vi "Stalled.vi"(6 "Stall Time (ms)":u32=300, 7 "Model Name":T1=enum."W 601 FR RH Std", 9 "Max Run Current":dbl=10.0, 10 "millisecond timer value in":u32, 11 "Inputs":T2) -> (1 "Stalled":bool, 2 "millisecond timer value out":u32)   [LabVIEW 2017]
uses:
  controls/All Inputs.ctl
  controls/SACB DI.ctl
  controls/Model Name.ctl
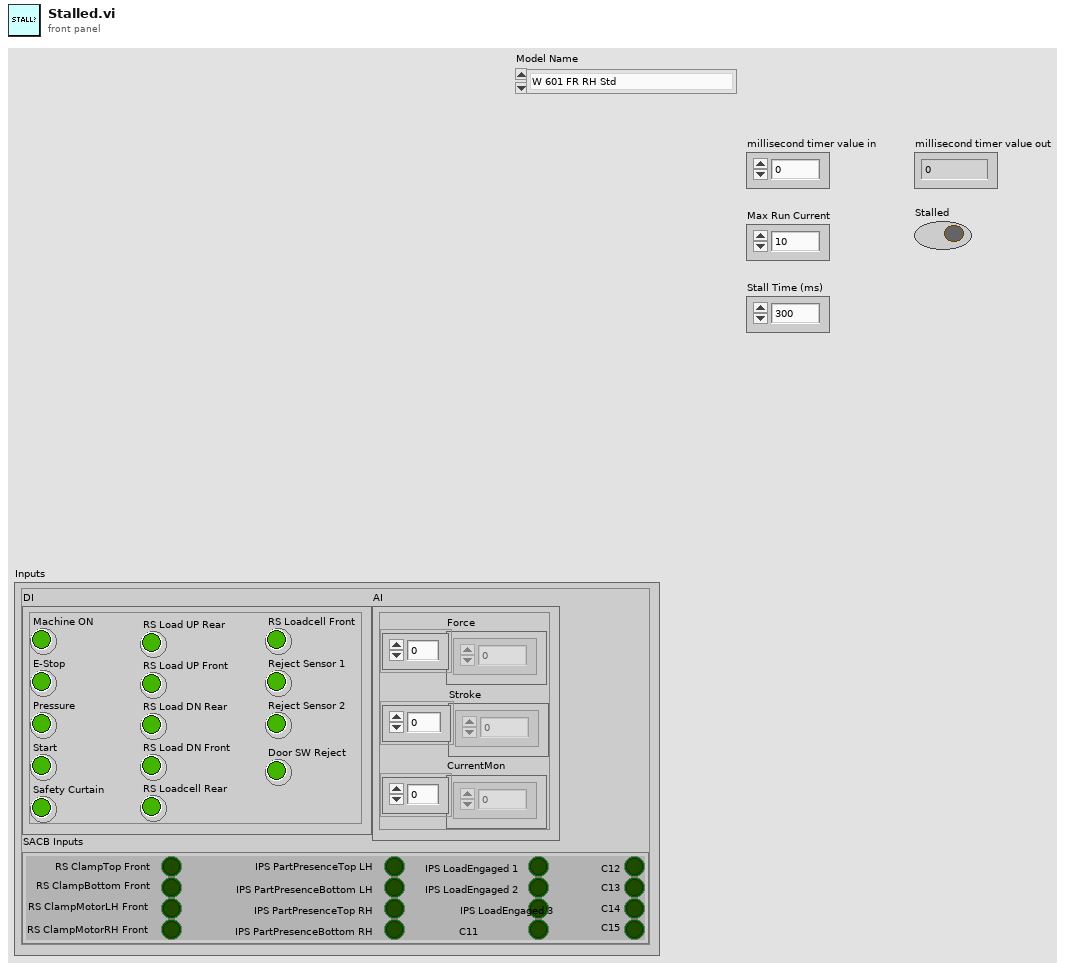
[diagram p1: front panel]
types:
  T1 = typedef "Model Name.ctl" = enum16{"W 501 FLH Std.", "W 501 FRH Std.", "W 601 FR RH Std", "W 601 FR LH Std", "W 601 RR RH Std", "W 601 RR LH Std", "W 601 FR RH AP", "W 601 FR LH AP", "W 601 RR RH AP", "W 601 RR LH AP"}
  T2 = typedef "All Inputs.ctl" = cluster{"DI":cluster{"Machine ON":bool, "E-Stop":bool, "Pressure":bool, "Start":bool, "Safety Curtain":bool, "RS Load UP Rear":bool, "RS Load UP Front":bool, "RS Load DN Rear":bool, "RS Load DN Front":bool, "RS Loadcell Rear":bool, "RS Loadcell Front":bool, "Reject Sensor 1":bool, "Reject Sensor 2":bool, "Door SW Reject":bool}, "AI":cluster{"Force":dbl[], "Stroke":dbl[], "CurrentMon":dbl[]}, "SACB Inputs":T3}
  T3 = typedef "SACB DI.ctl" = cluster{"RS ClampTop Front":bool, "RS ClampBottom Front":bool, "RS ClampMotorLH Front":bool, "RS ClampMotorRH Front":bool, "IPS PartPresenceTop LH":bool, "IPS PartPresenceBottom LH":bool, "IPS PartPresenceTop RH":bool, "IPS PartPresenceBottom RH":bool, "IPS LoadEngaged 1":bool, "IPS LoadEngaged 2":bool, "IPS LoadEngaged 3":bool, "C11":bool, "C12":bool, "C13":bool, "C14":bool, "C15":bool}
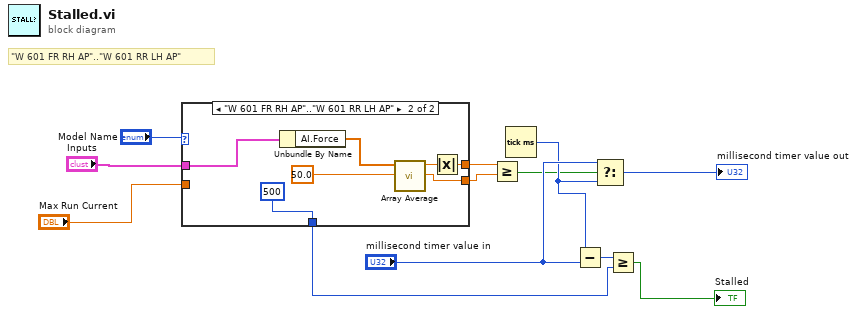
[diagram p0: block diagram]
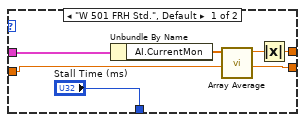
[diagram p2: hidden frame]
diagram:
  # "\"W 601 FR RH AP\"..\"W 601 RR LH AP\""
  n1 = case shown="\"W 601 FR RH AP\"..\"W 601 RR LH AP\"" "Model Name" {
    tunnel: [w16 w22] -> w6
    tunnel: "Inputs" -> [w15 w21]
    tunnel: [w14 50.0 ("Max Run Current 2")] -> w3
    tunnel: "Max Run Current" -> [w14 _]
    tunnel: ["Stall Time (ms)" u32 500 ("Stall Time (ms)")] -> w1
    frame "W 501 FRH Std.", Default {
      n2 = Unbundle By Name(w15) -> ("AI.CurrentMon"=w18:dbl[])
      n3 = call "Array Average.vi"("data"=w18) -> ("Numeric"=w17:dbl)  [unwired: 10 in]
      n4 = Absolute Value(x=w17) -> (abs(x)=w16:dbl)
    }
    frame "W 601 FR RH AP".."W 601 RR LH AP" {
      n5 = Unbundle By Name(w21) -> ("AI.Force"=w24:dbl[])
      n6 = call "Array Average.vi"("data"=w24) -> ("Numeric"=w23:dbl)  [unwired: 10 in]
      n7 = Absolute Value(x=w23) -> (abs(x)=w22:dbl)
    }
  }
  n8 = Greater Or Equal?(x=w6, y=w3) -> (x >= y?=w7:bool)
  n9 = Tick Count (ms)() -> (millisecond timer value=w9:u32)
  n10 = Subtract(x=w9, y="millisecond timer value in") -> (x-y=w11:u32)
  n11 = Select(t="millisecond timer value in", s=w7, f=w9) -> (s? t:f=→"millisecond timer value out":u32)
  n12 = Greater Or Equal?(x=w11, y=w1) -> (x >= y?=→"Stalled":bool)
